vi "Volt To physical quantity.vi"(6 "precision (6)":i16=3, 9 "Volt Input":dbl, 11 "Calibration":T1) -> (3 "physical quantity":dbl)   [LabVIEW 2017, in "SQLite.lvclass"]
doc: "Volt to physical quantity 根据不同的输入k b，得到相应的物理量。\n2015-05-29 15:53:39\n蒋松\njiangsong@outlook.com"
uses:
  SQLite.lvclass
  Calibration K and b.ctl
panel:
  out "x+y":dbl
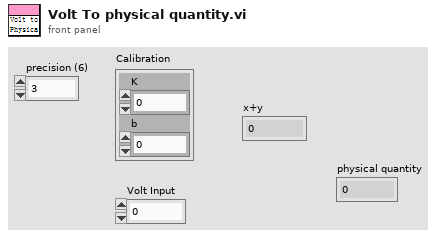
[diagram p1: front panel]
types:
  T1 = typedef "SQLite.lvclass/Calibration K and b.ctl" = cluster{"K":dbl, "b":dbl}
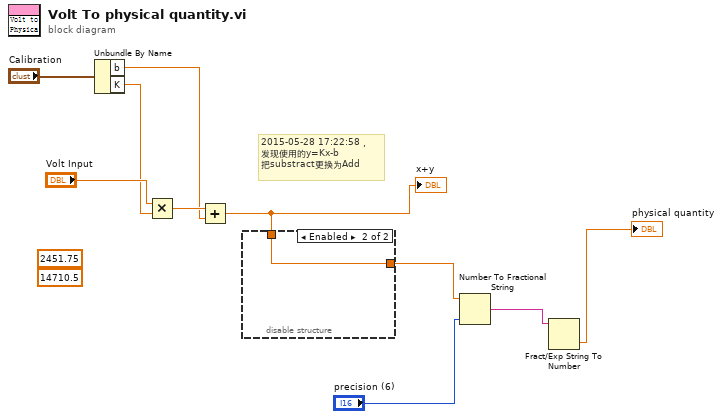
[diagram p0: block diagram]
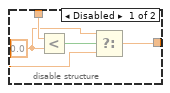
[diagram p2: hidden frame]
diagram:
  (unwired) 14710.5 ("y")
  (unwired) 2451.75 ("y")
  # "2015-05-28 17:22:58，\n发现使用的y=Kx-b\n把substract更换为Add"
  n1 = Unbundle By Name("Calibration") -> ("b"=w6:dbl, "K"=w7:dbl)
  n2 = Multiply(x="Volt Input", y=w7) -> (x*y=w9:dbl)
  n3 = Add(x=w9, y=w6) -> (x+y=w10:dbl)
  "x+y" <- w10
  n4 = disable-structure shown="Enabled" {
    disable-tunnel: [w14 w15] -> w2
    disable-tunnel: w10 -> [w13 w15]
    frame Disabled {
      w12 = 0.0 ("y")
      n5 = Less?(x=w13, y=w12) -> (x < y?=w11:bool)
      n6 = Select(t=w12, s=w11, f=w13) -> (s? t:f=w14:dbl)
    }
    frame Enabled {
    }
  }
  n7 = Number To Fractional String(number=w2, precision (6)="precision (6)") -> (F-format string=w5:string)  [unwired: 2 in]
  n8 = Fract/Exp String To Number(string=w5) -> (number=→"physical quantity":dbl)  [unwired: 3 in, 1 out]
